vi "in_Hermite interpolating polynomial.vi"(8 "index i":i32, 9 "Y deriv[0..N]":dbl[](array[numeric]) format="%_6g", 10 "X[0..N]":dbl[](array[numeric]) format="%_6g", 11 "Y[0..N]":dbl[](array[numeric]) format="%_6g") -> (3 "Hermite polynomial":dbl[](array[numeric]) format="%_6g")   [LabVIEW 2010, in "NI_Gmath.lvlib"]
uses:
  NI_Gmath.lvlib
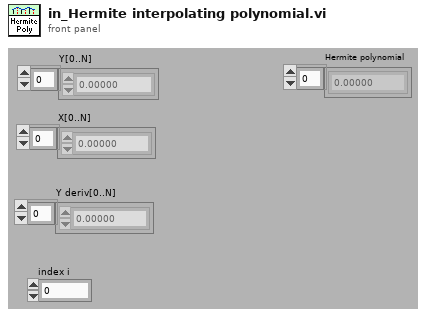
[diagram p1: front panel]
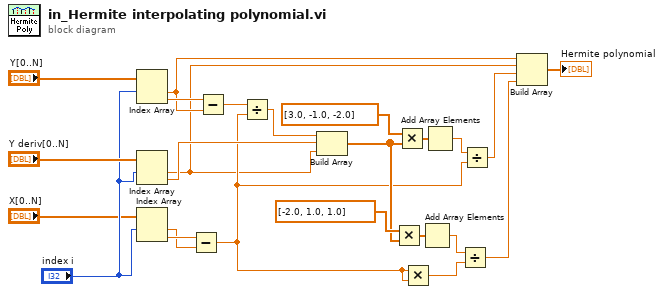
[diagram p0: block diagram]
diagram:
  n1 = Index Array(array="Y[0..N]", index #1="index i") -> (element #1=w6:dbl, element #2=w22:dbl)  [unwired: 1 in]
  n2 = Index Array(array="Y deriv[0..N]", index #1="index i") -> (element #1=w5:dbl, element #2=w16:dbl)  [unwired: 1 in]
  n3 = Index Array(array="X[0..N]", index #1="index i") -> (element #1=w17:dbl, element #2=w19:dbl)  [unwired: 1 in]
  n4 = Subtract(x=w19, y=w17) -> (x-y=w8:dbl)
  n5 = Subtract(x=w22, y=w6) -> (x-y=w21:dbl)
  n6 = Divide(x=w21, y=w8) -> (x/y=w1:dbl)
  n7 = Build Array(w1, w16, w5) -> (w11:dbl[])
  n8 = Multiply(x=dbl[] [-2.0, 1.0, 1.0], y=w11) -> (x*y=w13:dbl[])
  n9 = Multiply(x=dbl[] [3.0, -1.0, -2.0], y=w11) -> (x*y=w14:dbl[])
  n10 = Multiply(x=w8, y=w8) -> (x*y=w7:dbl)
  n11 = Add Array Elements(numeric array=w13) -> (sum=w9:dbl)
  n12 = Add Array Elements(numeric array=w14) -> (sum=w10:dbl)
  n13 = Divide(x=w9, y=w7) -> (x/y=w3:dbl)
  n14 = Divide(x=w10, y=w8) -> (x/y=w4:dbl)
  n15 = Build Array(w6, w5, w4, w3) -> (→"Hermite polynomial":dbl[])
